vi "Update Time.vi"(8 "error in (no error)":errorcluster, 11 "Timing Module in":refnum<class "Timing Module.lvclass">) -> (0 "error out":errorcluster, 3 "Timing Module out":refnum<class "Timing Module.lvclass">)   [LabVIEW 2020, in "Volatus.lvlib" / "Timing Module.lvclass"]
uses:
  Timing Module.lvclass
  Timing Module.lvclass/Timing Module.ctl
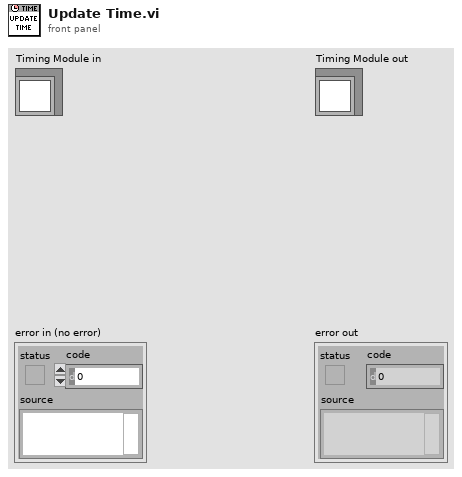
[diagram p1: front panel]
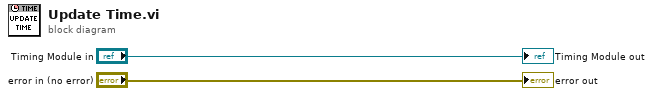
[diagram p0: block diagram]
diagram:
  "error out" <- "error in (no error)"
  "Timing Module out" <- "Timing Module in"
